vi "Read list and Write Headers to Excel Summary File.vi"(8 "error in":errorcluster, 9 "Headers Path":path=path "C:/ModisEdge/Scope/Test Sequence/Headers_ModisEdge.ini", 10 "summary file prefix":string="MES_Test Results_", 11 "data base path":path=path "C:/Snap-On/ModisEdgeScope") -> (0 "error out":errorcluster, 1 "Excel column headers":string[](array[string])=["Test Date", "Time", "SN", "Station ID", "Overall Pass/Fail Results", "(0.0) +3.3V Voltage Test", "(0.1) +5.2V Voltage Test", "(0.2) +5.2VA Voltage Test", "(0.3) -5.2VA Voltage Test", "(0.4) +1.6V Voltage Test", "Initialize Calibration Table - MEScope_CalStructInit", "1.0 Get DSP Version", "1.1 Get Firmware Version", "1.2 Test Silo Memory", "( 1.3 - 1.9 ) Load Data Registers", "(2.0) ToggleACTestMode", "(2.1) Zero Calibrate all channels", "(3.0) Calibrate 1 Volt", "(3.1) Calibrate 2 Volts", "(3.2) Calibrate 5 Volts", "(3.3) Calibrate 10 Volts", "(3.4) Calibrate 20 Volts", "(3.5) Calibrate 50 Volts", "(3.6) Calibrate 100 Volts", "(3.7) Calibrate 200 Volts", "(3.8) Calibrate 400 Volts", "(4.0) Calibrate Zero Ohms", "(4.1) Calibrate 40 Ohms", "(4.2) Calibrate 400 Ohms", "(4.3) Calibrate 4k Ohms", "(4.4) Calibrate 40k Ohms", "(4.5) Calibrate 400k Ohms", "(4.6) Calibrate 4M Ohms", "CalStruct_IncrementNumCals", "Calstruct_Write", "Calstruct_Read", "Calstruct View", "Calstruct_Read Second time", "Calstruct View", "Compare Tables", "(5.0) Verify 0.5V Cal for Ch1", "(5.1) Verify 0.5V Cal for Ch2", "(5.2) Verify +1.0V Cal for Ch1", "(5.3) Verify +1.0V Cal for Ch2", "(5.4) Verify +2.5V Cal for Ch1", "(5.5) Verify +2.5V Cal for Ch2", "(5.6) Verify +5.0V Cal for Ch1", "(5.7) Verify +5.0V Cal for Ch2", "(5.8) Verify +10V Cal for Ch1", "(5.9) Verify +10V Cal for Ch2", "(5.10) Verify +25V Cal for Ch1", "(5.11) Verify +25V Cal for Ch2", "(5.12) Verify +50V Cal for Ch1", "(5.13) Verify +50V Cal for Ch2", "(5.14) Verify +100V Cal for Ch1", "(5.15) Verify +100V Cal for Ch2", "(5.16) Verify +200V Cal for Ch1", "(5.17) Verify +200V Cal for Ch2", "(6.1) AC Coupling Test on CH1", "(6.2) AC Coupling Test on CH2", "(7.1) AC Response Test on Ch1", "(7.2) AC Response Test on Ch2", "(8.1) Verify 0 Ohms 40 Ohms scale", "(8.2) Verify 0 Ohms 400 Ohms scale", "(8.3) Verify 0 Ohms 4k Ohms scale", "(8.4) Verify 0 Ohms 40k Ohms scale", "(8.5) Verify 0 Ohms 400k Ohms scale", "(8.6) Verify 0 Ohms 4Meg Ohms scale", "(8.7) Verify 20 Ohms 40 Ohms scale", "(8.8) Verify 200 Ohms 400 Ohms scale", "(8.9) Verify 2k Ohms 4k Ohms scale", "(8.10) Verify 20k Ohms 40k Ohms scale", "(8.11) Verify 200k Ohms 400k Ohms scale", "(8.12) Verify 2Meg Ohms 4Meg Ohms scale"], 2 "start cell":cluster{"row":i32, "column":i32}={"row"=1, "column"=0}, 3 "summary file path":path=path "C:/Snap-On/ModisEdgeScope/TabletScope Test Results_2016-04.xlsx")   [LabVIEW 2015]
uses:
  <vilib>/addons/_office/excel.llb/Excel Get Data ([str]).vi
  <vilib>/Utility/NIReport.llb/NI_report.lvclass
  <vilib>/Utility/NIReport.llb/Excel/NI_Excel.lvclass
  <vilib>/addons/_office/NI_ReportGenerationToolkit.lvlib
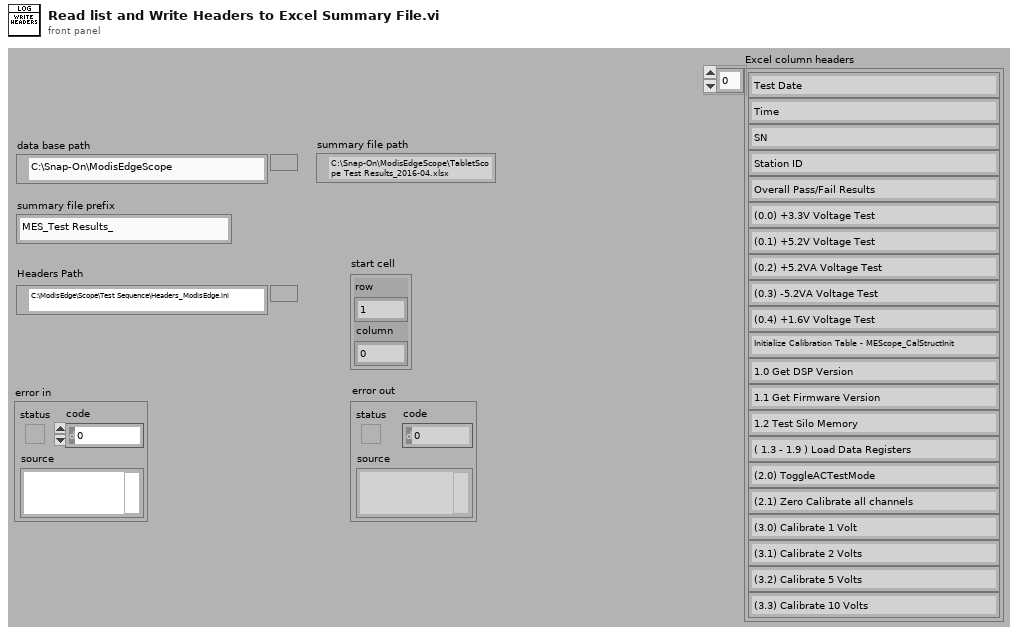
[diagram p1: front panel]
types:
  T1 = enum16{"maximized", "minimized", "normal", "no change"}
  T2 = enum16{"Standard Report", "HTML", "Word", "Excel"}
  T3 = cluster{"position (Excel)":cluster{"row":i32, "column":i32}, "name (Excel)":string, "bookmark (Word)":string}
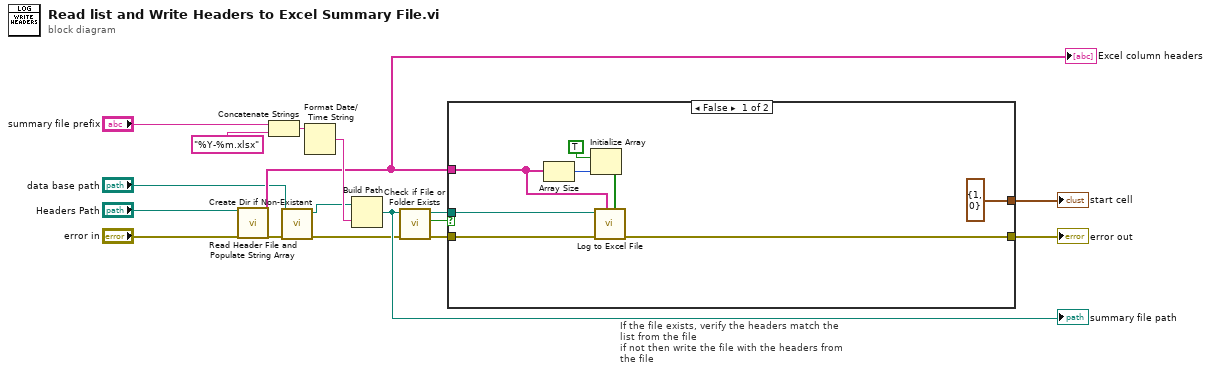
[diagram p0: block diagram]
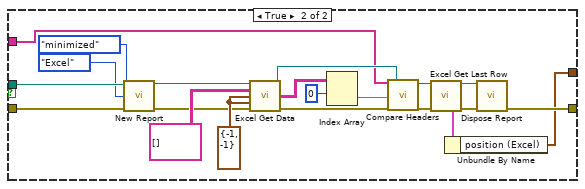
[diagram p2: hidden frame]
diagram:
  n1 = call "Read Header File and Populate String Array.vi"("file path (dialog if empty)"="Headers Path", "error in (no error)"="error in") -> ("subarray"=w5:string[], "error out"=w3:errorcluster)  [unwired: 16 in]
  "Excel column headers" <- w5
  n2 = Concatenate Strings("summary file prefix", "%Y-%m.xlsx" ("time format string (%c)")) -> (w13:string)
  n3 = call "Create Dir if Non-Existant.vi"("error in (no error)"=w3, "Directory Path"="data base path") -> ("error out"=w8:errorcluster, "dup Directory Path"=w7:path)  [unwired: 7 in, 1 out]
  n4 = Format Date/Time String(time format string (%c)=w13) -> (date/time string=w17:string)  [unwired: 2 in]
  n5 = Build Path(base path=w7, name or relative path=w17) -> (appended path=w15:path)
  "summary file path" <- w15
  n6 = call <vilib>:"Check if File or Folder Exists.vi"("error in (no error)"=w8, "path"=w15) -> ("error out"=w10:errorcluster, "file or folder exists?"=w11:bool, "dup path"=w16:path)  [unwired: 7 in]
  n7 = case "If the file exists, verify the headers match the list from the file\nif not then write the file with the headers from the file" shown="False" w11 {
    tunnel: w16 -> [w20 w45]
    tunnel: w5 -> [w22 w27]
    tunnel: [w19 w41] -> w9
    tunnel: w10 -> [w24 w37]
    tunnel: [cluster{"row":i32, "column":i32} {"row"=1, "column"=0} ("position (Excel)") w38] -> w6
    frame False {
      n8 = Array Size(array=w22) -> (size(s)=w23:i32)
      n9 = Initialize Array(TRUE, w23) -> (w21:bool[])
      n10 = call "Log to Excel File.vi"("status"=w21, "data"=w22, "error in"=w24, "report file path"=w20) -> ("error out"=w19:errorcluster)  [unwired: 6 in, 1 out]
    }
    frame True {
      w35 = cluster{"row":i32, "column":i32} {"row"=-1, "column"=-1} ("start (-1, -1)")
      n11 = call <vilib>:"New Report.vi"("window state (normal)"=T1."minimized", "report type"=T2."Excel", "template (empty)"=w45, "error in (no error)"=w37) -> ("report out"=w31:refnum<class "NI_report.lvclass">, "error out"=w34:errorcluster)  [unwired: 10 in]
      n12 = call-poly <vilib>:"Excel Get Data.vi"("report in"=w31, "data type"=string[][] [], "start (-1, -1)"=w35, "end (-1, -1)"=w35, "error in (no error)"=w34) -> ("report out"=w30:refnum<class "NI_report.lvclass">, "data"=w33:string[][], "error out"=w29:errorcluster)  [unwired: 8 in]
      n13 = Index Array(array=w33, index (row)=0) -> (element=w26:string[])  [unwired: 1 in]
      n14 = call "Compare Headers.vi"("Headers From File"=w27, "Current Headers"=w26, "error in (no error)"=w29) -> ("error out"=w28:errorcluster)  [unwired: 16 in]
      n15 = call <vilib>:"Excel Get Last Row.vi"("report in"=w30, "error in (no error)"=w28) -> ("report out"=w40:refnum<class "NI_report.lvclass">, "MS Office parameters out"=w39:T3, "error out"=w42:errorcluster)  [unwired: 11 in]
      n16 = Unbundle By Name(w39) -> ("position (Excel)"=w38:cluster{"row":i32, "column":i32})
      n17 = call-dynamic "Dispose Report.vi"("report in"=w40, "error in (no error)"=w42) -> ("error out"=w41:errorcluster)  [unwired: 13 in]
    }
  }
  "error out" <- w9
  "start cell" <- w6
